vi "Launch Forecast Data Actor.vi"(8 "error in":errorcluster, 11 "SCADA in":refnum<class "EMS.lvclass">) -> (0 "error out":errorcluster, 3 "SCADA out":refnum<class "EMS.lvclass">)   [LabVIEW 2018, in "EMS Core.lvlib" / "EMS.lvclass"]
uses:
  EMS.lvclass
  C:/Users/Administrator/Desktop/LabVIEW EMS/EMS Generic Actor/EMS Generic/EMS Generic.lvclass
  C:/Program Files (x86)/National Instruments/LabVIEW 2018/vi.lib/ActorFramework/Actor/Actor.lvclass
  IED Actors/ForecastData Actor/ForecastData/ForecastData.lvclass
  <vilib>/ORNL/CSEISMIC DDS/CSEISMIC DDS Base/Data Types/Controls/DeviceClass Selector.ctl
  EMS.lvclass/EMS.ctl
  <vilib>/ActorFramework/Actor/Actor.lvclass
  <vilib>/ORNL/CSEISMIC DDS/CSEISMIC DDS Base/CSEISMIC DDS.lvclass
  EMS Generic Actor/EMS Generic/EMS Generic.lvclass
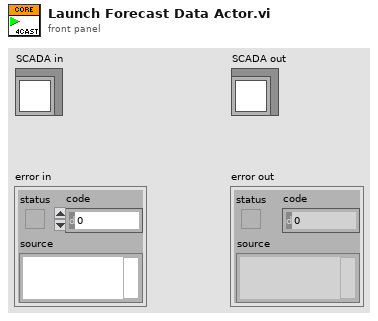
[diagram p1: front panel]
types:
  T1 = typedef "CSEISMIC DDS.lvlib/CSEISMIC DDS.lvclass/DeviceID.ctl" = string
  T2 = typedef "CSEISMIC DDS.lvlib/CSEISMIC DDS.lvclass/DeviceClass Selector.ctl" = u16
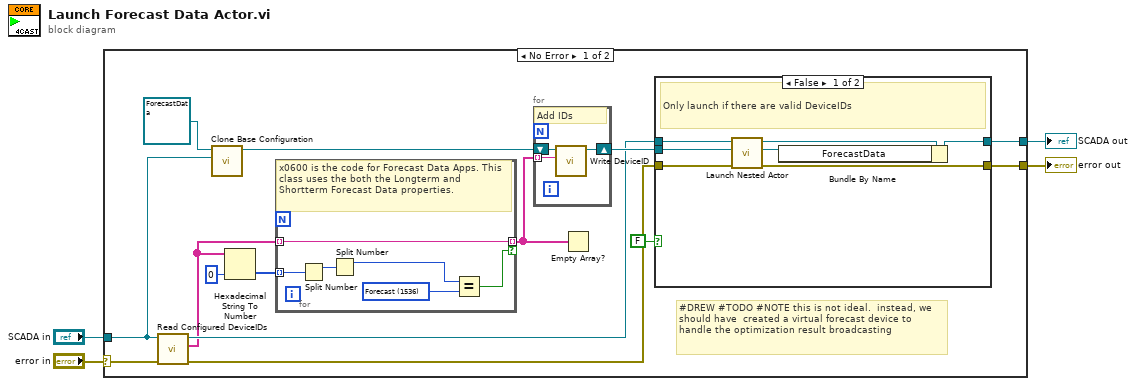
[diagram p0: block diagram]
diagram:
  n1 = case shown="No Error" "error in" {
    selector: "error in" -> [w9 w38]
    tunnel: [w17 w38] -> w3
    tunnel: [w18 w37] -> w1
    tunnel: "SCADA in" -> [w6 w37]
    frame No Error {
      # "#DREW #TODO #NOTE this is not ideal.  instead, we should have  created a virtual forecast device to handle the optimization result broadcasting"
      n2 = call "Read Configured DeviceIDs.vi"("error in"=w9, "EMS Generic in"=w6) -> ("error out"=w13:errorcluster, "DeviceIDs"=w11:T1[], "EMS Generic out"=w14:refnum<class "EMS.lvclass">)  [unwired: 7 in]
      n3 = call-dynamic "Clone Base Configuration.vi"("Source Object"=w6, "Target Object in"=refnum<class "ForecastData.lvclass"> refnum ("ForecastData Actor.lvlib:ForecastData.lvclass")) -> ("Target Object out"=w7:refnum<class "ForecastData.lvclass">)  [unwired: 9 in]
      n4 = Hexadecimal String To Number(string=w11, default (0uL)=u64 0 ("default (0 U32)")) -> (number=w10:u64[])  [unwired: 1 in, 1 out]
      n5 = for {
        tunnel: w11 -> [w34] mode=indexing
        tunnel: [w34] -> w15 mode=indexing if=w33
        tunnel: w10 -> [w31] mode=indexing
        w32 = T2 1536 items=["Invalid"=0, "IED"=256, "DER"=512, "Relay"=768, "Meter"=1024, "Load"=1280, "Forecast"=1536, "Price"=1792, "Energy Storage"=513, "PV"=514, "Generator"=515, "Smart Relay"=769, "PCC"=770, "Smart Meter"=1025, "PMU"=1026, "HVAC"=1281] ("DeviceClass")
        # "x0600 is the code for Forecast Data Apps. This class uses the both the Longterm and Shortterm Forecast Data properties."
        n6 = Split Number(x=w31) -> (hi(x)=w36:u32)  [unwired: 1 out]
        n7 = Split Number(x=w36) -> (hi(x)=w35:u16)  [unwired: 1 out]
        n8 = Equal?(x=w35, y=w32) -> (x = y?=w33:bool)
      }
      n9 = for {
        shift-right: [w29] -> w16
        shift-left: w7 -> [w30]
        tunnel: w15 -> [w28] mode=indexing
        # "Add IDs"
        n10 = call-dynamic "Write DeviceID.vi"("DeviceID"=w28, "Device DDS Communications in"=w30) -> ("Device DDS Communications out"=w29:refnum<class "ForecastData.lvclass">)  [unwired: 9 in]
      }
      n11 = Empty Array?(array=w15) -> ()  [unwired: 1 out]
      n12 = case shown="False" FALSE {
        tunnel: [w20 w27] -> w18
        tunnel: w13 -> [w24 w26]
        tunnel: [w23 w26] -> w17
        tunnel: w16 -> [w22 _]
        tunnel: w14 -> [w21 w27]
        frame False {
          # "Only launch if there are valid DeviceIDs"
          n13 = call <vilib>:"Launch Nested Actor.vi"("error in (no error)"=w24, "Nested Actor"=w22, "Caller Actor in"=w21) -> ("error out"=w23:errorcluster, "Nested Actor's Enqueuer"=w19:refnum<class "Message Enqueuer.lvclass">, "Caller Actor out"=w25:refnum<class "EMS.lvclass">)  [unwired: 6 in]
          n14 = Bundle By Name(cluster=w25, "ForecastData"=w19) -> (w20:refnum<class "EMS.lvclass">)
        }
        frame True {
        }
      }
    }
    frame Error {
    }
  }
  "error out" <- w3
  "SCADA out" <- w1
